vi "FormLogin.vi"() -> ()   [LabVIEW 2013]
uses:
  <vilib>/addons/database/_DB Variant To Data/Database Variant To Data.xnode
panel:
  out "管理员":string(combo)
  out "编号":string(combo)
  in  "联机模式":enum32{"未选择", "联网模式", "单机模式"}(radio)
  in  "用户登录":bool
  out "udl名称":string="epsacc.udl"
  in  "修改密码":bool
  in  "用户名":string(combo)
  in  "密码":string
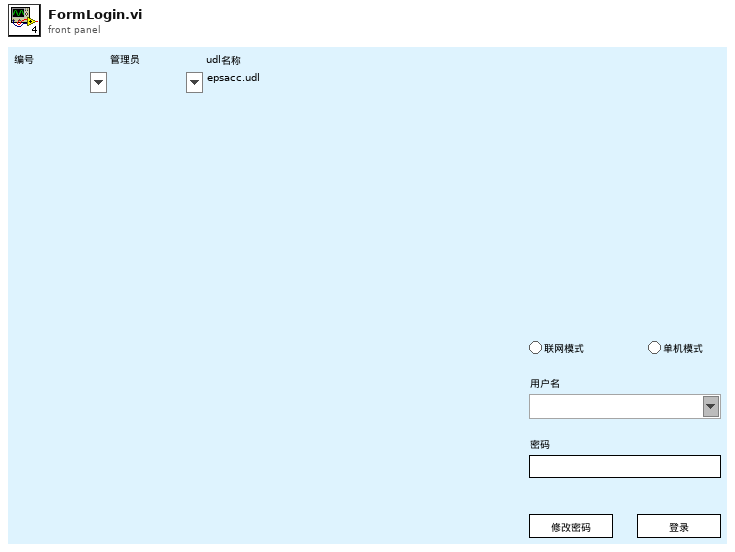
[diagram p1: front panel]
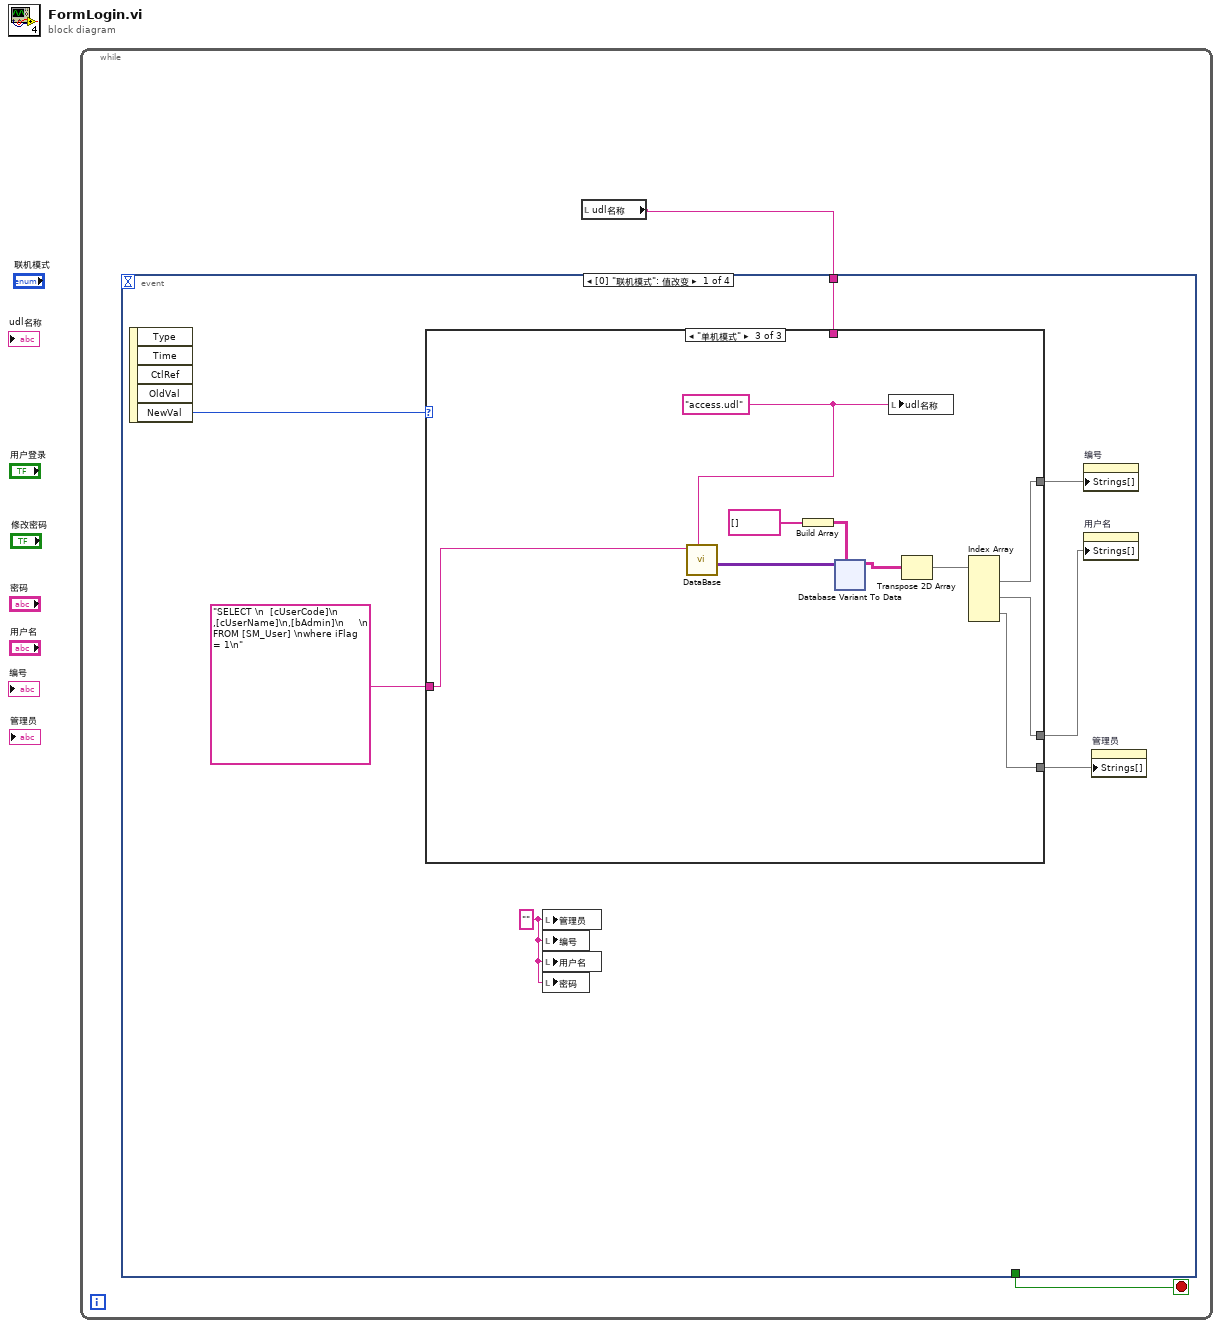
[diagram p0: block diagram]
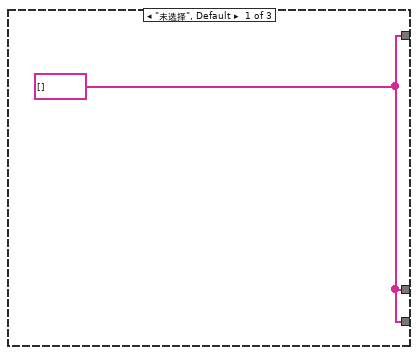
[diagram p2: hidden frame]
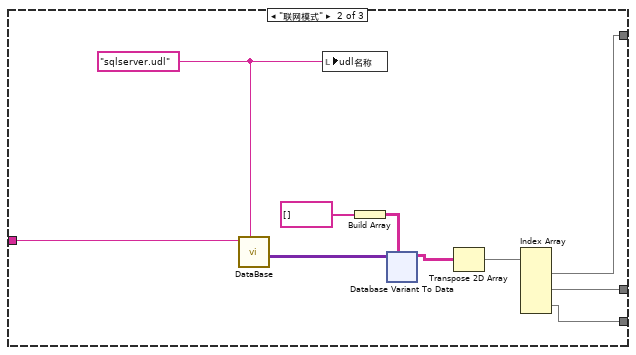
[diagram p3: hidden frame]
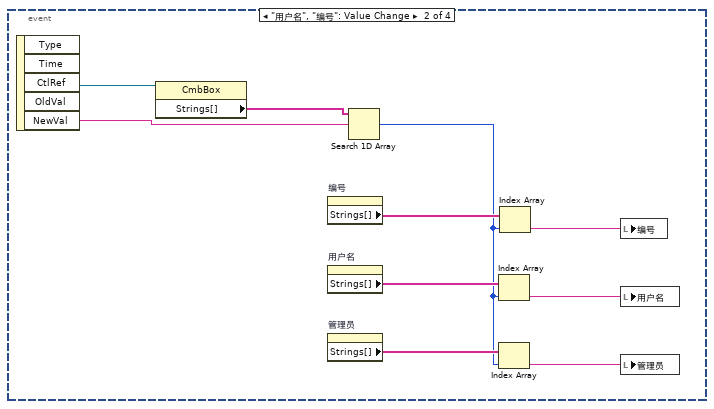
[diagram p4: hidden frame]
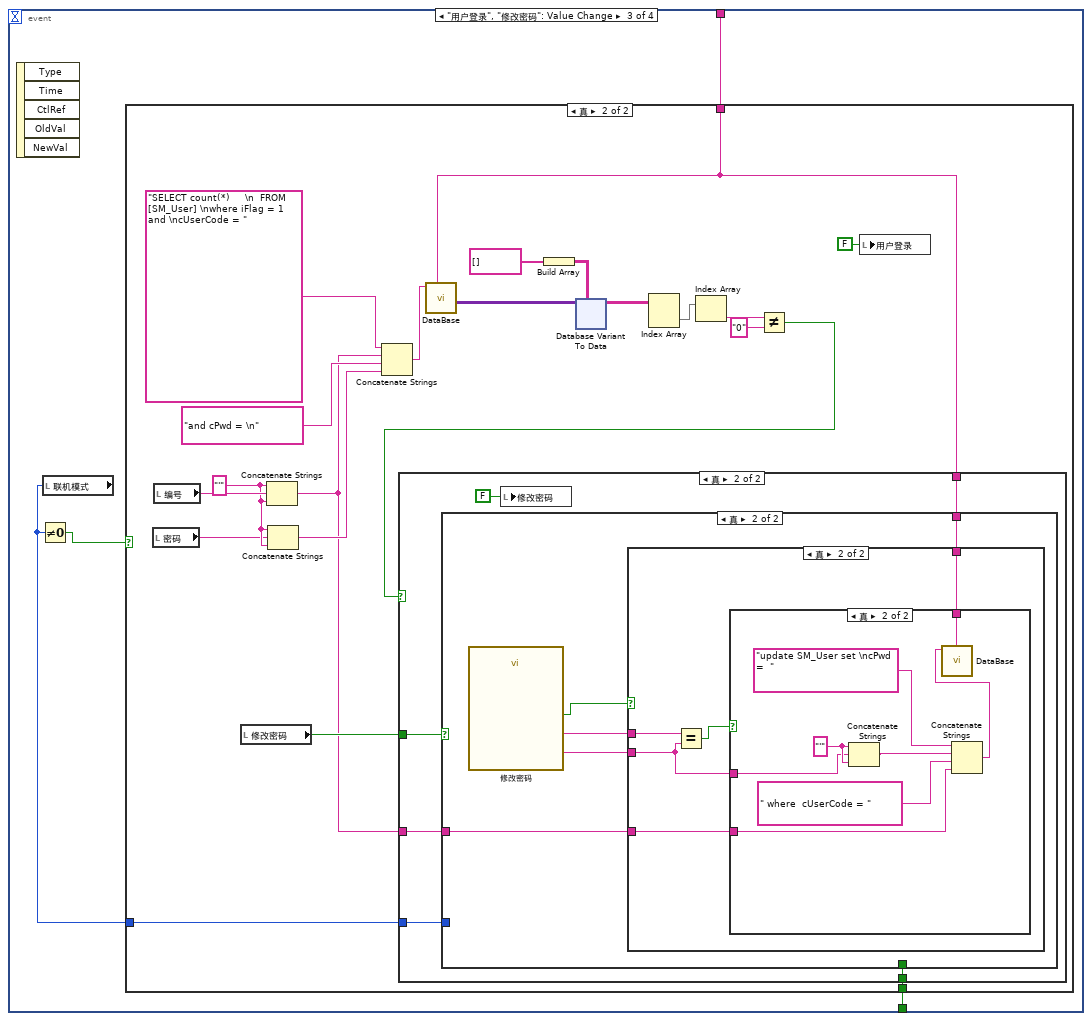
[diagram p5: hidden frame]
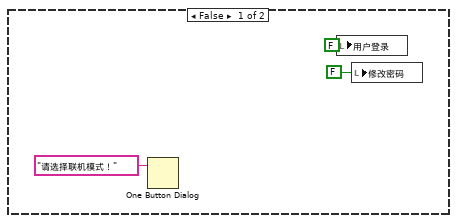
[diagram p6: hidden frame]
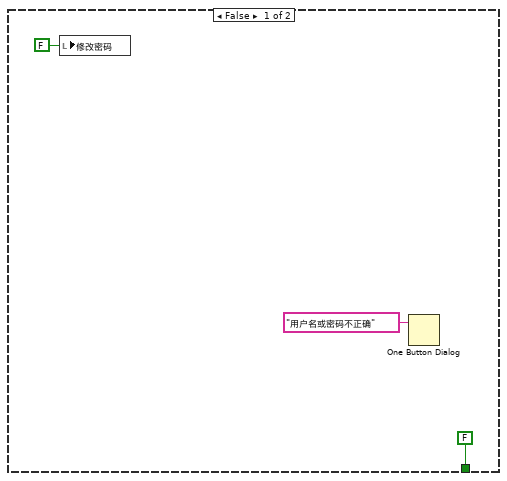
[diagram p7: hidden frame]
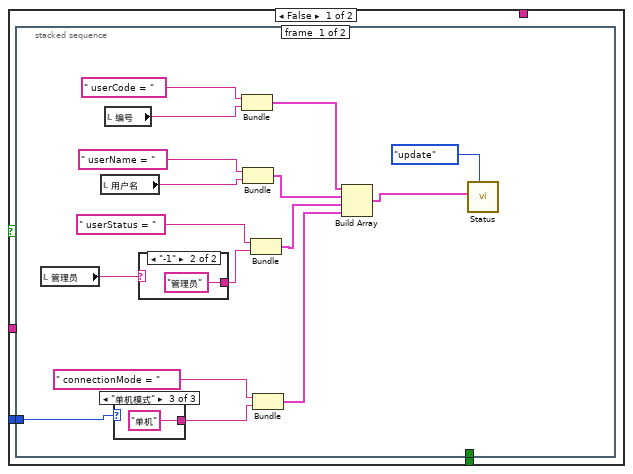
[diagram p8: hidden frame]
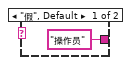
[diagram p9: hidden frame]
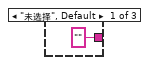
[diagram p10: hidden frame]
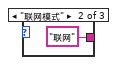
[diagram p11: hidden frame]
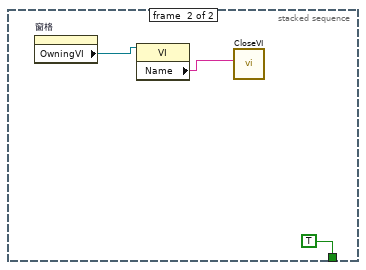
[diagram p12: hidden frame]
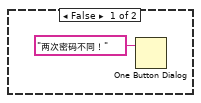
[diagram p14: hidden frame]
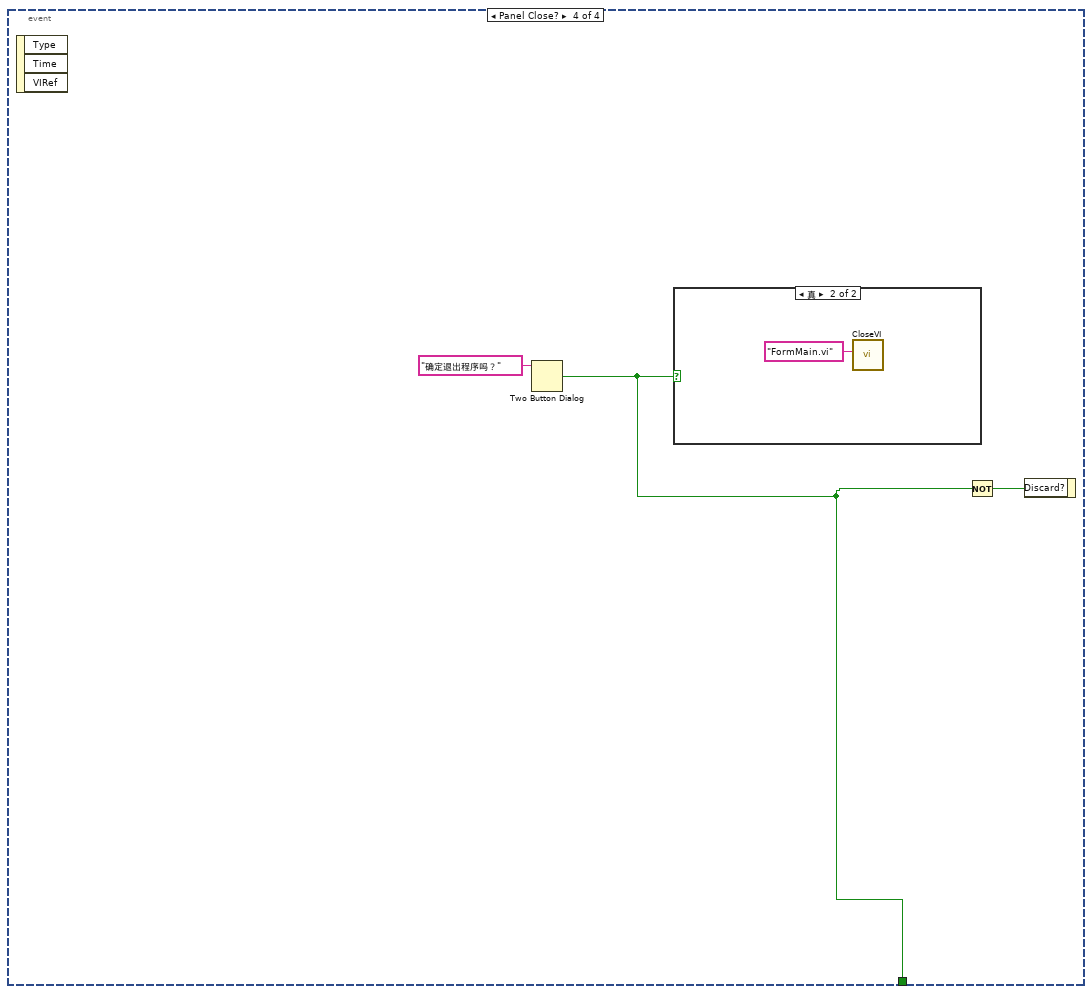
[diagram p15: hidden frame]
diagram:
  n1 = while {
    stop <- w2 stop-if-true
    n2 = local read "udl名称"() -> (w1:string)
    n3 = event shown="[0] \"联机模式\": 值改变" {
      selector: _ -> [_ _ _ _]
      dyn-events: _ -> [_ _ _ _]
      timeout: _ -> [_ _ _ _]
      tunnel: [_ _ w132 w255] -> w2
      tunnel: w1 -> [w8 _ w131 _]
      event "联机模式": Value Change {
        w3 = "" ("密码")
        n4 = event-data() -> ("NewVal"=w9:enum32{"未选择", "联网模式", "单机模式"})  [unwired: 1 in, 4 out]
        n5 = case shown="\"单机模式\"" w9 {
          tunnel: w8 -> [_ _ _]
          tunnel: [w10 w14 w69] -> w7
          tunnel: "SELECT \n  [cUserCode]\n     ,[cUserName]\n,[bAdmin]\n     \n  FROM [SM_User] \nwhere iFlag = 1\n" ("SQL query") -> [_ w13 w67]
          tunnel: [w10 w12 w66] -> w5
          tunnel: [w10 w11 w65] -> w4
          frame "未选择", Default {
            w10 = string[] [] ("字符串[]")
          }
          frame "联网模式" {
            w15 = "sqlserver.udl" ("udl名称")
            n6 = call "DataBase.vi"("udl名称"=w15, "SQL query"=w13) -> ("recordset data"=w17:variant[][])  [unwired: 9 in]
            n7 = local write "udl名称"(w15) -> ()
            n8 = Build Array(string[] [] ("添加的数组")) -> (w19:string[][])
            n9 = xnode "Database Variant To Data"("database variant"=w17, "type"=w19) -> ("data"=w18:string[][])  [unwired: 1 in, 1 out]
            n10 = Transpose 2D Array(2D array=w18) -> (transposed array=w16:string[][])
            n11 = Index Array(array=w16) -> (element #1=w14:string[], element #2=w12:string[], element #3=w11:string[])  [unwired: 6 in]
          }
          frame "单机模式" {
            w68 = "access.udl" ("udl名称")
            n12 = call "DataBase.vi"("udl名称"=w68, "SQL query"=w67) -> ("recordset data"=w71:variant[][])  [unwired: 9 in]
            n13 = Build Array(string[] [] ("添加的数组")) -> (w73:string[][])
            n14 = xnode "Database Variant To Data"("database variant"=w71, "type"=w73) -> ("data"=w72:string[][])  [unwired: 1 in, 1 out]
            n15 = local write "udl名称"(w68) -> ()
            n16 = Transpose 2D Array(2D array=w72) -> (transposed array=w70:string[][])
            n17 = Index Array(array=w70) -> (element #1=w69:string[], element #2=w66:string[], element #3=w65:string[])  [unwired: 6 in]
          }
        }
        n18 = local write "管理员"(w3) -> ()
        n19 = local write "编号"(w3) -> ()
        n20 = local write "用户名"(w3) -> ()
        n21 = local write "密码"(w3) -> ()
        n22 = property on="编号" class="CmbBox"("Strings[]"=w7) -> ()  [unwired: 2 in, 2 out]
        n23 = property on="用户名" class="CmbBox"("Strings[]"=w5) -> ()  [unwired: 2 in, 2 out]
        n24 = property on="管理员" class="CmbBox"("Strings[]"=w4) -> ()  [unwired: 2 in, 2 out]
      }
      event "用户名", "编号": Value Change {
        n25 = event-data() -> ("CtlRef"=w128:refnum<vi>, "NewVal"=w126:string)  [unwired: 1 in, 3 out]
        n26 = property class="CmbBox"(reference=w128) -> ("Strings[]"=w127:string[])  [unwired: 1 in, 2 out]
        n27 = property on="编号" class="CmbBox"() -> ("Strings[]"=w125:string[])  [unwired: 2 in, 2 out]
        n28 = property on="用户名" class="CmbBox"() -> ("Strings[]"=w124:string[])  [unwired: 2 in, 2 out]
        n29 = property on="管理员" class="CmbBox"() -> ("Strings[]"=w120:string[])  [unwired: 2 in, 2 out]
        n30 = Search 1D Array(1D array=w127, element=w126) -> (index of element=w119:i32)  [unwired: 1 in]
        n31 = Index Array(array=w124, index=w119) -> (element=w122:string)
        n32 = Index Array(array=w120, index=w119) -> (element=w121:string)
        n33 = Index Array(array=w125, index=w119) -> (element=w123:string)
        n34 = local write "编号"(w123) -> ()
        n35 = local write "用户名"(w122) -> ()
        n36 = local write "管理员"(w121) -> ()
      }
      event "用户登录", "修改密码": Value Change {
        n37 = event-data() -> ()  [unwired: 1 in, 5 out]
        n38 = local read "联机模式"() -> (w129:enum32{"未选择", "联网模式", "单机模式"})
        n39 = Not Equal To 0?(x=w129) -> (x != 0?=w130:bool)
        n40 = case shown="真" w130 {
          tunnel: [_ w156] -> w132
          tunnel: w131 -> [_ w136]
          tunnel: w129 -> [_ w138]
          frame False {
            n41 = One Button Dialog(message="请选择联机模式！" ("消息")) -> ()  [unwired: 1 in, 1 out]
            n42 = local write "用户登录"(FALSE ("登录")) -> ()
            n43 = local write "修改密码"(FALSE ("登录")) -> ()
          }
          frame True {
            w151 = "'"
            n44 = local read "密码"() -> (w150:string)
            n45 = local read "编号"() -> (w152:string)
            n46 = local read "修改密码"() -> (w144:bool)
            n47 = Concatenate Strings(w151, w152, w151) -> (w137:string)
            n48 = Concatenate Strings(w151, w150, w151) -> (w147:string)
            n49 = Concatenate Strings("SELECT count(*)     \n  FROM [SM_User] \nwhere iFlag = 1 and \ncUserCode = " ("SQL query"), w137, "and cPwd = \n" ("SQL query"), w147) -> (w146:string)
            n50 = call "DataBase.vi"("udl名称"=w136, "SQL query"=w146) -> ("recordset data"=w153:variant[][])  [unwired: 9 in]
            n51 = Build Array(string[] [] ("添加的数组")) -> (w154:string[][])
            n52 = xnode "Database Variant To Data"("database variant"=w153, "type"=w154) -> ("data"=w145:string[][])  [unwired: 1 in, 1 out]
            n53 = Index Array(array=w145) -> (element=w143:string[])  [unwired: 2 in]
            n54 = Index Array(array=w143) -> (element=w142:string)  [unwired: 1 in]
            n55 = Not Equal?(x=w142, y="0") -> (x != y?=w140:bool)
            n56 = case shown="真" w140 {
              tunnel: [FALSE w209] -> w156
              tunnel: w144 -> [_ w208]
              tunnel: w138 -> [_ w206]
              tunnel: w137 -> [_ w205]
              tunnel: w136 -> [_ w204]
              frame False {
                n57 = local write "修改密码"(FALSE ("登录")) -> ()
                n58 = One Button Dialog(message="用户名或密码不正确" ("消息")) -> ()  [unwired: 1 in, 1 out]
              }
              frame True {
                n59 = case shown="真" w208 {
                  tunnel: [w211 _] -> w209
                  tunnel: w206 -> [w210 _]
                  tunnel: w205 -> [_ w237]
                  tunnel: w204 -> [_ w236]
                  frame False {
                    n60 = stacked-sequence {
                      tunnel: [_ TRUE] -> w211
                      tunnel: w210 -> [w227 _]
                      frame #0 {
                        n61 = local read "管理员"() -> (w226:string)
                        n62 = local read "用户名"() -> (w222:string)
                        n63 = local read "编号"() -> (w224:string)
                        n64 = case shown="\"单机模式\"" w227 {
                          tunnel: ["" "联网" "单机"] -> w219
                          frame "未选择", Default {
                          }
                          frame "联网模式" {
                          }
                          frame "单机模式" {
                          }
                        }
                        n65 = case shown="\"-1\"" w226 {
                          tunnel: ["操作员" "管理员"] -> w221
                          frame "假", Default {
                          }
                          frame "-1" {
                          }
                        }
                        n66 = Bundle("y"=" userCode = ", "编号"=w224) -> (w217:cluster{"y":string, "编号":string})  [unwired: 1 in]
                        n67 = Bundle("y"=" userName = ", "用户名"=w222) -> (w216:cluster{"y":string, "用户名":string})  [unwired: 1 in]
                        n68 = Bundle("y"=" userStatus = ", w221) -> (w215:cluster{"y":string, string})  [unwired: 1 in]
                        n69 = Bundle("y"=" connectionMode = ", w219) -> (w214:cluster{"y":string, string})  [unwired: 1 in]
                        n70 = Build Array(w217, w216, w215, w214) -> (w212:cluster{"y":string, "用户名":string}[])
                        n71 = call "Status.vi"("模式"=enum16{"select", "insert", "update", "delete"}."update", "nameData"=w212) -> ()  [unwired: 9 in, 1 out]
                      }
                      frame #1 {
                        n72 = property on="窗格" class="Pane"() -> ("OwningVI"=w234:refnum<vi>)  [unwired: 2 in, 2 out]
                        n73 = property class="VI"(reference=w234) -> ("Name"=w233:string)  [unwired: 1 in, 2 out]
                        n74 = call "CloseVI.vi"("名称或相对路径"=w233) -> ()  [unwired: 10 in, 1 out]
                      }
                    }
                  }
                  frame True {
                    n75 = call "修改密码"() -> ("确认密码"=w238:string, "新密码"=w239:string, "确定"=w240:bool)  [unwired: 16 in, 1 out]
                    n76 = case shown="真" w240 {
                      tunnel: w239 -> [_ w245]
                      tunnel: w238 -> [_ w242]
                      tunnel: w236 -> [_ w243]
                      tunnel: w237 -> [_ w241]
                      frame False {
                      }
                      frame True {
                        n77 = Equal?(x=w245, y=w242) -> (x = y?=w244:bool)
                        n78 = case shown="真" w244 {
                          tunnel: w243 -> [_ w254]
                          tunnel: w242 -> [_ w247]
                          tunnel: w241 -> [_ w251]
                          frame False {
                            n79 = One Button Dialog(message="两次密码不同！" ("消息")) -> ()  [unwired: 1 in, 1 out]
                          }
                          frame True {
                            w249 = "'"
                            n80 = Concatenate Strings(w249, w247, w249) -> (w248:string)
                            n81 = Concatenate Strings("update SM_User set \ncPwd =  " ("SQL query"), w248, " where  cUserCode = " ("SQL query"), w251) -> (w250:string)
                            n82 = call "DataBase.vi"("udl名称"=w254, "SQL query"=w250) -> ()  [unwired: 9 in, 1 out]
                          }
                        }
                      }
                    }
                  }
                }
                n83 = local write "修改密码"(FALSE ("登录")) -> ()
              }
            }
            n84 = local write "用户登录"(FALSE ("登录")) -> ()
          }
        }
      }
      event Panel Close? {
        n85 = event-data() -> ()  [unwired: 1 in, 3 out]
        n86 = Two Button Dialog(message="确定退出程序吗？" ("消息")) -> (T button?=w255:bool)  [unwired: 2 in]
        n87 = case shown="真" w255 {
          frame False {
          }
          frame True {
            n88 = call "CloseVI.vi"("名称或相对路径"="FormMain.vi") -> ()  [unwired: 10 in, 1 out]
          }
        }
        n89 = Not(x=w255) -> (.not. x?=w256:bool)
        n90 = event-data("Discard?"=w256) -> ()  [unwired: 1 in, 1 out]
      }
    }
  }
